vi "Post Error.vi"(4 "Post \"No error\" Message to SysLog if No Error (T)":bool=TRUE, 6 "Clear Incoming Error (T)":bool=TRUE, 8 "Error In":errorcluster, 10 "Message":string, 11 "Custom Device Name":string) -> (0 "Error Out":errorcluster, 1 "Error Code":i32)   [LabVIEW 2018]
doc: "Use this VI to post errors and warnings to the System Log and to write the error code to the custom device's <B>Status.Error Code</B> channel.\n\nIf your custom device is writing more data to your output FIFO, you may use this VI to post the error/warning to the System Log and to retrieve the error code that can be inserted into your FIFO values array at the appropriate index.\n\nThis VI is reentrant. It stores the previous error value and compares it to the current error value to determine if the error condition has recently been cleared. If desired, the VI can post a \"No error\" message to the System Log when the previous error condition is cleared."
uses:
  <vilib>/Utility/SystemLogging/NI_SystemLogging.lvlib
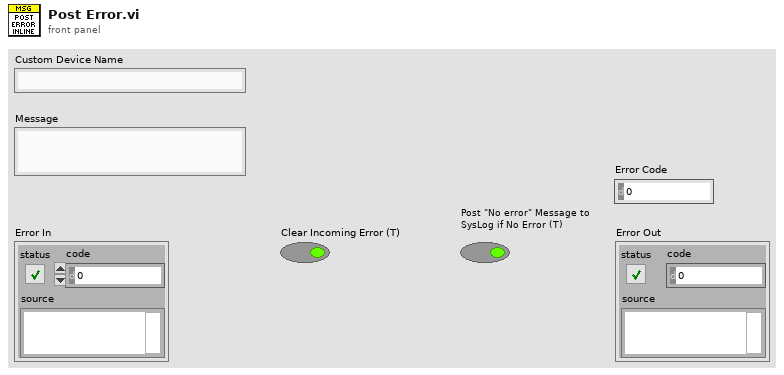
[diagram p1: front panel]
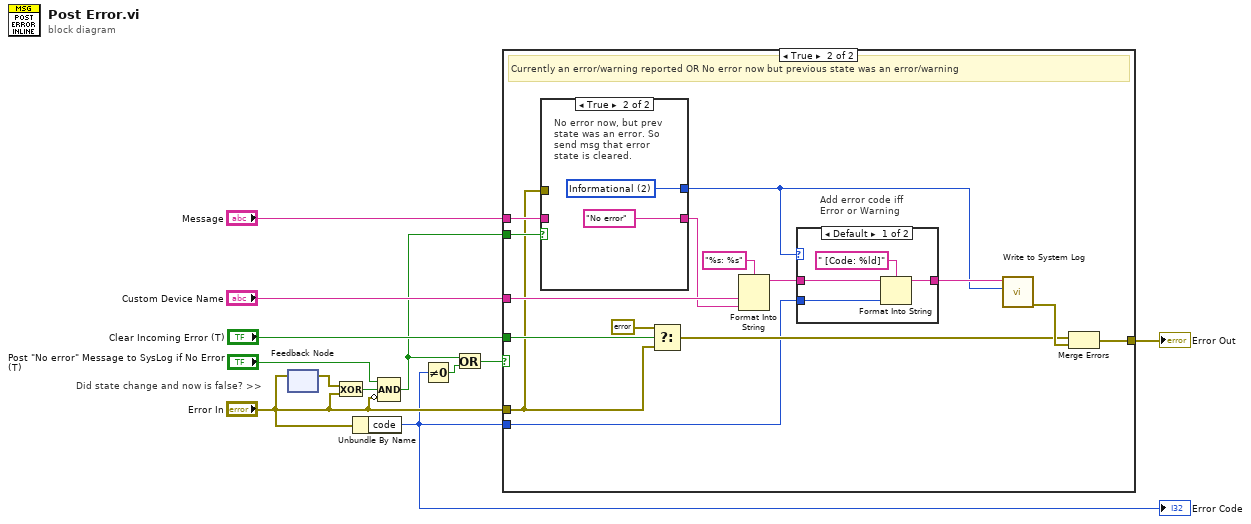
[diagram p0: block diagram]
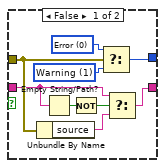
[diagram p3: hidden frame]
diagram:
  # "Did state change and now is false? >>"
  n1 = feedback #1() -> (w8:errorcluster)  [unwired: 1 in]
  n2 = feedback-in #1("Error In") -> ()
  n3 = Exclusive Or(1:"Error In", 2:w8) -> (0:w7:bool)
  n4 = Unbundle By Name("Error In") -> ("code"=w1:i32)
  "Error Code" <- w1
  n5 = Compound Arithmetic op=AND("Post \"No error\" Message to SysLog if No Error (T)", w7, invert "Error In") -> (w4:bool)
  n6 = Not Equal To 0?(x=w1) -> (x != 0?=w5:bool)
  n7 = Or(x=w4, y=w5) -> (x .or. y?=w2:bool)
  n8 = case shown="True" w2 {
    tunnel: "Custom Device Name" -> [_ w27]
    tunnel: "Clear Incoming Error (T)" -> [_ w21]
    tunnel: [w13 w20] -> w10
    tunnel: "Message" -> [_ w17]
    tunnel: w4 -> [_ w16]
    tunnel: "Error In" -> [w13 w15]
    tunnel: w1 -> [_ w14]
    frame False {
      # "No current error/warning reported AND Previous state was not an error/warning"
    }
    frame True {
      # "Add error code iff Error or Warning"
      # "Currently an error/warning reported OR No error now but previous state was an error/warning"
      n9 = case shown="True" w16 {
        tunnel: [w35 w39] -> w18
        tunnel: [w30 "No error" ("format string")] -> w19
        tunnel: w17 -> [w29 _]
        tunnel: w15 -> [w34 _]
        frame False {
          w37 = 0 items=["Error", "Warning", "Informational"] ("severity")
          w36 = 1 items=["Error", "Warning", "Informational"] ("severity")
          n10 = Unbundle By Name(w34) -> ("source"=w31:string)
          n11 = Empty String/Path?(string/path=w29) -> (empty?=w33:bool)
          n12 = Not(x=w33) -> (.not. x?=w32:bool)
          n13 = Select(t=w37, s=w34, f=w36) -> (s? t:f=w35:i32)
          n14 = Select(t=w29, s=w32, f=w31) -> (s? t:f=w30:string)
        }
        frame True {
          w39 = 2 items=["Error", "Warning", "Informational"] ("severity")
          # "No error now, but prev state was an error. So send msg that error state is cleared."
        }
      }
      n15 = Select(t=errorcluster {"status"=FALSE, "code"=0, "source"=""}, s=w21, f=w15) -> (s? t:f=w23:errorcluster)
      n16 = Format Into String(format string="%s: %s", w27, w19) -> (resulting string=w26:string)  [unwired: 2 in, 1 out]
      n17 = case shown="Default" w18 {
        tunnel: w26 -> [w43 w44]
        tunnel: w14 -> [w41 _]
        tunnel: [w40 w44] -> w25
        frame Default {
          n18 = Format Into String(format string=" [Code: %ld]", initial string=w43, w41) -> (resulting string=w40:string)  [unwired: 1 in, 1 out]
        }
        frame 2 {
        }
      }
      n19 = call <vilib>:"Write to System Log.vi"("severity"=w18, "message"=w25) -> ("error out"=w24:errorcluster)  [unwired: 9 in]
      n20 = Merge Errors(w23, w24) -> (w20:errorcluster)
    }
  }
  "Error Out" <- w10
